vi "FlatToRichniswitch_grpc_ConnectRequest.vi"(5 "OutputClusterType":T1, 11 "InputCluster":T3) -> (3 "OutputCluster":T1)   [LabVIEW 2021, in "NI Switch_client.lvlib"]
uses:
  NI Switch_client.lvlib
  nidevice_grpc_Session.ctl
  niswitch_grpc_ConnectRequest.ctl
  nidevice_grpc_Session_Flat.ctl
  niswitch_grpc_ConnectRequest_Flat.ctl
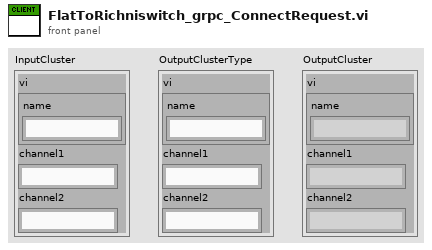
[diagram p1: front panel]
types:
  T1 = typedef "NI Switch_client.lvlib/niswitch_grpc_ConnectRequest.ctl" = cluster{"vi":T2, "channel1":string, "channel2":string}
  T2 = typedef "NI Switch_client.lvlib/nidevice_grpc_Session.ctl" = cluster{"name":string}
  T3 = typedef "NI Switch_client.lvlib/niswitch_grpc_ConnectRequest_Flat.ctl" = cluster{"vi":T4, "channel1":string, "channel2":string}
  T4 = typedef "NI Switch_client.lvlib/nidevice_grpc_Session_Flat.ctl" = cluster{"name":string}
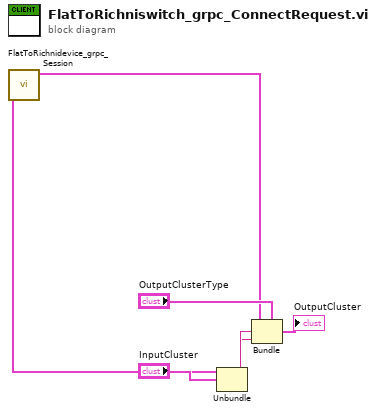
[diagram p0: block diagram]
diagram:
  n1 = Unbundle "Unbundle"("InputCluster") -> ("vi"=w4:T4, "channel1"=w2:string, "channel2"=w1:string)
  n2 = call "FlatToRichnidevice_grpc_Session.vi"("InputCluster"=w4) -> ("OutputCluster"=w3:T2)  [unwired: 10 in]
  n3 = Bundle "Bundle"(cluster="OutputClusterType", "vi"=w3, "channel1"=w2, "channel2"=w1) -> (→"OutputCluster":T1)
